vi "Write 2D Double Array as Numpy.vi"(3 "error in":errorcluster, 4 "Array":dbl[][](array[numeric]), 5 "Path":path) -> (0 "error out":errorcluster)   [LabVIEW 2013, in "PyLab.lvlib"]
uses:
  PyLab.lvlib
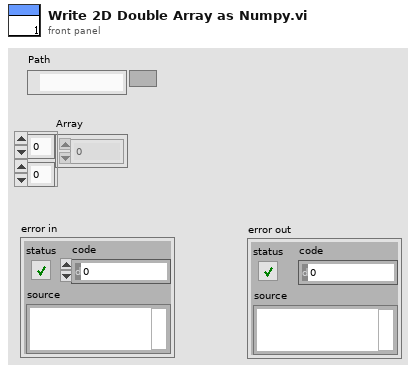
[diagram p1: front panel]
types:
  T1 = enum16{"big-endian, network order", "native, host order", "little-endian"}
  T2 = enum16{"open", "replace", "create", "open or create", "replace or create", "replace or create with confirmation"}
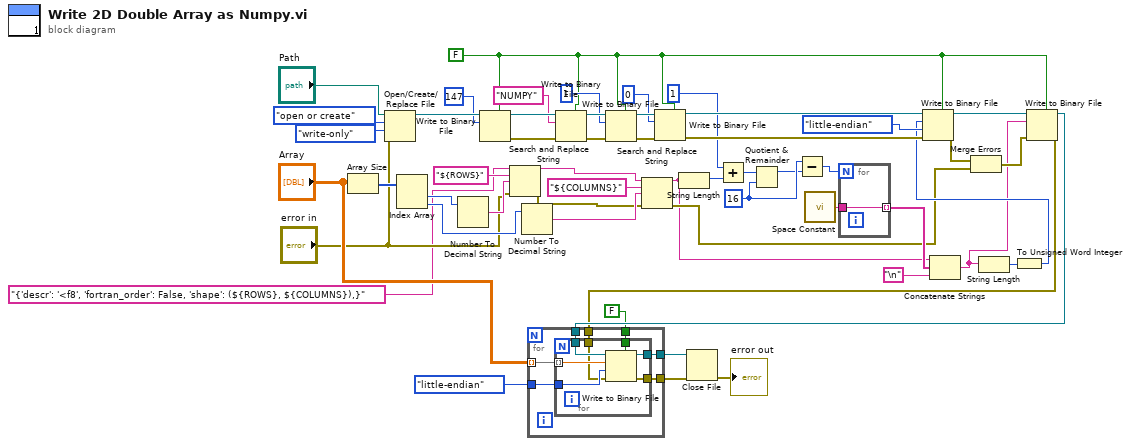
[diagram p0: block diagram]
diagram:
  w20 = FALSE ("prepend array or string size? (T)")
  w7 = u16 16
  n1 = Array Size(array="Array") -> (size(s)=w36:i32[])
  n2 = Open/Create/Replace File(file path (use dialog)="Path", error in="error in", operation (0:open)=T2."open or create", access (0:read/write)=enum16{"read/write", "read-only", "write-only"}."write-only") -> (refnum out=w51:refnum<file>)  [unwired: 2 in, 2 out]
  n3 = Index Array(array=w36) -> (element #1=w35:i32, element #2=w32:i32)  [unwired: 2 in]
  n4 = Number To Decimal String(number=w35) -> (decimal integer string=w14:string)  [unwired: 1 in]
  n5 = Write to Binary File(file (use dialog)=w51, data=u8 147, 5:w20) -> (refnum out=w48:refnum<file>, error out=w49:errorcluster)  [unwired: 3 in, 1 out]
  n6 = Search and Replace String(input string="{'descr': '<f8', 'fortran_order': False, 'shape': (${ROWS}, ${COLUMNS}),}", search string="${ROWS}", replace string=w14, error in="error in") -> (result string=w33:string, error out=w12:errorcluster)  [unwired: 4 in, 2 out]
  n7 = Number To Decimal String(number=w32) -> (decimal integer string=w31:string)  [unwired: 1 in]
  n8 = Write to Binary File(file (use dialog)=w48, data="NUMPY", error in=w49, 5:w20) -> (refnum out=w45:refnum<file>, error out=w46:errorcluster)  [unwired: 2 in, 1 out]
  n9 = Write to Binary File(file (use dialog)=w45, data=u8 1 ("Numeric"), error in=w46, 5:w20) -> (refnum out=w42:refnum<file>, error out=w43:errorcluster)  [unwired: 2 in, 1 out]
  n10 = Search and Replace String(input string=w33, search string="${COLUMNS}", replace string=w31, error in=w12) -> (result string=w8:string, error out=w10:errorcluster)  [unwired: 4 in, 2 out]
  n11 = Write to Binary File(file (use dialog)=w42, data=u8 0, error in=w43, 5:w20) -> (refnum out=w39:refnum<file>, error out=w40:errorcluster)  [unwired: 2 in, 1 out]
  n12 = String Length(string=w8) -> (length=w29:i32)
  n13 = Add(x=u16 1, y=w29) -> (x+y=w26:i32)
  n14 = Quotient & Remainder(x=w26, y=w7) -> (x-y*floor(x/y)=w6:i32)  [unwired: 1 out]
  n15 = Subtract(x=w7, y=w6) -> (x-y=w5:i32)
  n16 = call <vilib>:"Space Constant.vi"() -> ("String"=w28:string)
  n17 = for {
    N: w5 -> [_]
    tunnel: w28 -> [w55]
    tunnel: [w55] -> w27 mode=indexing
  }
  n18 = Concatenate Strings(w8, w27, "\n") -> (w4:string)
  n19 = String Length(string=w4) -> (length=w3:i32)
  n20 = To Unsigned Word Integer(number=w3) -> (unsigned 16bit integer=w25:u16)
  n21 = Write to Binary File(file (use dialog)=w39, data=w25, error in=w40, 5:w20, 9:T1."little-endian" ("byte order (0:big-endian, network order)")) -> (refnum out=w24:refnum<file>, error out=w11:errorcluster)  [unwired: 1 in, 1 out]
  n22 = Merge Errors(w11, w10) -> (w9:errorcluster)
  n23 = Write to Binary File(file (use dialog)=w24, data=w4, error in=w9, 5:w20) -> (refnum out=w22:refnum<file>, error out=w18:errorcluster)  [unwired: 2 in, 1 out]
  n24 = for {
    tunnel: "Array" -> [w62] mode=indexing
    tunnel: w22 -> [w61]
    tunnel: FALSE ("prepend array or string size? (T)") -> [w60]
    tunnel: T1."little-endian" ("byte order (0:big-endian, network order)") -> [w59]
    tunnel: w18 -> [w58]
    tunnel: [w57] -> w17
    tunnel: [w56] -> w16
    n25 = for {
      tunnel: w62 -> [w69] mode=indexing
      tunnel: w61 -> [w68]
      tunnel: w60 -> [w67]
      tunnel: w59 -> [w66]
      tunnel: w58 -> [w65]
      tunnel: [w64] -> w57
      tunnel: [w63] -> w56
      n26 = Write to Binary File(file (use dialog)=w68, data=w69, error in=w65, 5:w67, 9:w66) -> (refnum out=w63:refnum<file>, error out=w64:errorcluster)  [unwired: 1 in, 1 out]
    }
  }
  n27 = Close File(refnum=w16, error in=w17) -> (error out=→"error out":errorcluster)  [unwired: 1 out]
